vi "Single Acquisition.vi"() -> (3 "Out":fxp<+/-,12,12>)   [LabVIEW 2014]
doc: "Performs a single acquisition from DIO 0 to DIO 11 and returns a 12-bit FXD with integer word lenght 5-bit"
uses:
  <vilib>/rvi/eio/common/nirviEmuTemplateMethod_errors.vi
  <vilib>/eio/EIONode/EIONode.xnode
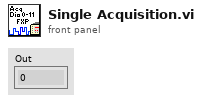
[diagram p1: front panel]
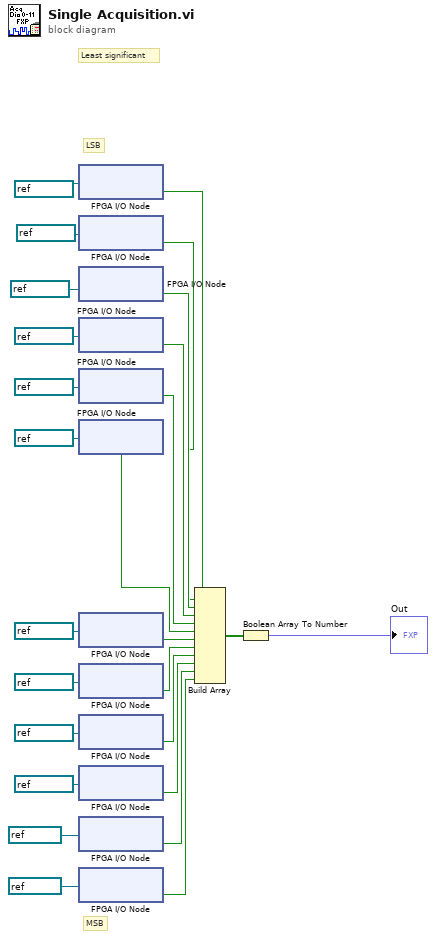
[diagram p0: block diagram]
diagram:
  # "MSB"
  # "LSB"
  # "Least significant"
  n1 = xnode "FPGA I/O Node"("FPGA I/O In"=refnum<k21> "DIO18") -> ("I/O Item"=w4:bool)  [unwired: 1 out]
  n2 = xnode "FPGA I/O Node"("FPGA I/O In"=refnum<k21> "DIO19") -> ("I/O Item"=w3:bool)  [unwired: 1 out]
  n3 = xnode "FPGA I/O Node"("FPGA I/O In"=refnum<k21> "DIO20") -> ("I/O Item"=w6:bool)  [unwired: 1 out]
  n4 = xnode "FPGA I/O Node"("FPGA I/O In"=refnum<k21> "DIO21") -> ("I/O Item"=w5:bool)  [unwired: 1 out]
  n5 = xnode "FPGA I/O Node"("FPGA I/O In"=refnum<k21> "DIO22") -> ("I/O Item"=w24:bool)  [unwired: 1 out]
  n6 = xnode "FPGA I/O Node"("FPGA I/O In"=refnum<k21> "DIO23") -> ("I/O Item"=w23:bool)  [unwired: 1 out]
  n7 = xnode "FPGA I/O Node"("FPGA I/O In"=refnum<k21> "DIO24") -> ("I/O Item"=w22:bool)  [unwired: 1 out]
  n8 = xnode "FPGA I/O Node"("FPGA I/O In"=refnum<k21> "DIO25") -> ("I/O Item"=w21:bool)  [unwired: 1 out]
  n9 = xnode "FPGA I/O Node"("FPGA I/O In"=refnum<k21> "DIO26") -> ("I/O Item"=w20:bool)  [unwired: 1 out]
  n10 = xnode "FPGA I/O Node"("FPGA I/O In"=refnum<k21> "DIO27") -> ("I/O Item"=w19:bool)  [unwired: 1 out]
  n11 = xnode "FPGA I/O Node"("FPGA I/O In"=refnum<k21> "DIO3") -> ("I/O Item"=w18:bool)  [unwired: 1 out]
  n12 = xnode "FPGA I/O Node"("FPGA I/O In"=refnum<k21> "DIO2") -> ("I/O Item"=w17:bool)  [unwired: 1 out]
  n13 = Build Array(w4, w3, w6, w5, w24, w23, w22, w21, w20, w19, w18, w17) -> (w2:bool[])
  n14 = Boolean Array To Number(Boolean array=w2) -> (number=→"Out":fxp<+/-,12,12>)
